vi "LineFollowerPID.vi"   [LabVIEW 2016, in "LineFollower2Sensor.lvrbt"]
uses:
  LineFollower2Sensor.lvrbt
  <vilib>/NXT/Block Support/NXT_InputPort.ctl
  <vilib>/NXT/Hardware/Plugins/Tetrix DC Motor/TetrixDCMotorAddress.ctl
  <vilib>/NXT/Dual Mode Library/Sensors/Light_On.vi
  <vilib>/NXT/NXTIO Xnodes/NXTIONodeSubVIs/TETRIX IO Move DC Motors.vi
  <vilib>/NXT/NXTIO Xnodes/AddressXNode/NXTIOAddress.xnode
  <vilib>/NXT/NXTIO Xnodes/NXTIOXNode/NXTIO.xnode
  <vilib>/NXT/Subs/LVHSConnector.ctl
  <vilib>/NXT/LegoClasses/BrickReference/BrickReference.lvclass
types:
  T1 = typedef "NXT_InputPort.ctl" = u32
  T2 = typedef "LVHSConnector.ctl" = refnum<class "BrickReference.lvclass">
  T3 = typedef "TetrixDCMotorAddress.ctl" = i32
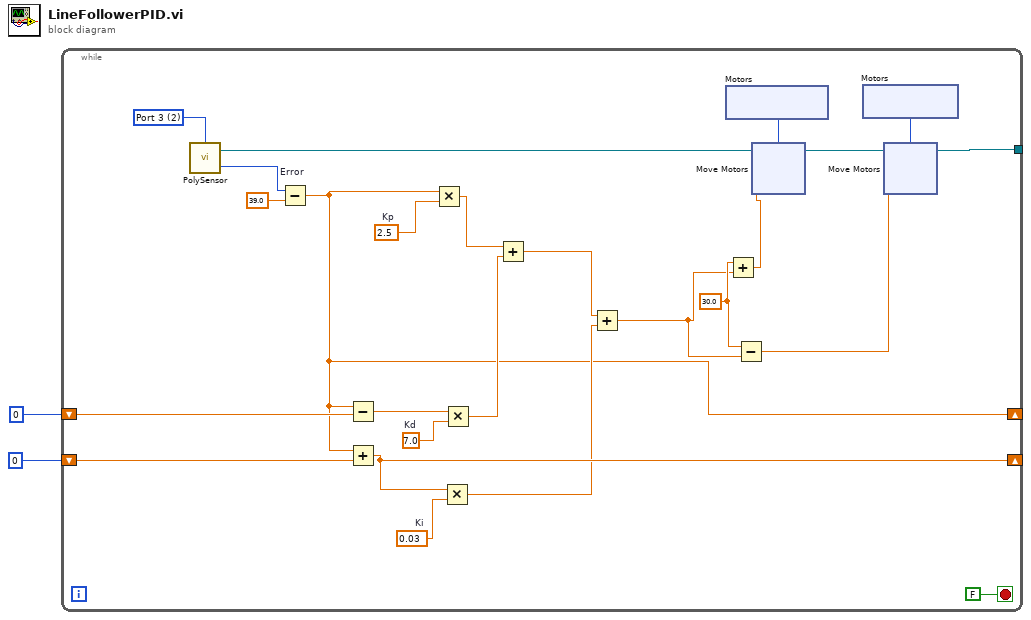
[diagram p0: block diagram]
diagram:
  n1 = while {
    shift-right: [w3] -> _
    shift-left: 0 -> [w21]
    shift-right: [w18] -> _
    shift-left: 0 -> [w20]
    tunnel: [w10] -> _
    stop <- FALSE stop-if-true
    w7 = 30.0 ("x")
    w17 = 7.0  # Kd
    w19 = 0.03  # Ki
    w23 = 2.5  # Kp
    w26 = T1 2 items=["Port 1", "Port 2", "Port 3", "Port 4"] ("Port (Port 3)")
    n2 = call-poly <vilib>:"PolySensor.vi"("Port (Port 3)"=w26) -> ("Scaled Value"=w24:i16, "NXT/EV3"=w12:T2)  [unwired: 2 in]
    n3 = Subtract "Error"(x=w24, y=39.0) -> (x-y=w3:dbl)
    n4 = Subtract(x=w3, y=w21) -> (x-y=w16:dbl)
    n5 = Add(x=w3, y=w20) -> (x+y=w18:dbl)
    n6 = Multiply(x=w3, y=w23) -> (x*y=w22:dbl)
    n7 = Multiply(x=w18, y=w19) -> (x*y=w14:dbl)
    n8 = Multiply(x=w16, y=w17) -> (x*y=w15:dbl)
    n9 = Add(x=w22, y=w15) -> (x+y=w13:dbl)
    n10 = Add(x=w13, y=w14) -> (x+y=w6:dbl)
    n11 = xnode "Motors"() -> ("Motor"=w8:T3)
    n12 = Add(x=w7, y=w6) -> (x+y=w4:dbl)
    n13 = Subtract(x=w7, y=w6) -> (x-y=w5:dbl)
    n14 = xnode "Move Motors"("Power/Speed 1"=w4, "Motors"=w8, "NXT/EV3"=w12) -> ("NXT/EV3"=w11:T2)
    n15 = xnode "Motors"() -> ("Motor"=w9:T3)
    n16 = xnode "Move Motors"("Power/Speed 1"=w5, "Motors"=w9, "NXT/EV3"=w11) -> ("NXT/EV3"=w10:T2)
  }
